vi "Get_Set_Timer_Parameters.vi"(6 "Get/Set":T2, 7 "Element":T3=enum."Current time", 8 "Status/Errors in":refnum<vi>, 9 "Timer parameters in":refnum<vi>, 10 "Value in":u32) -> (0 "Status/Errors out":refnum<vi>, 1 "Timer parameters out":refnum<vi>, 2 "Value out":u32, 3 "Timer cluster":T1={"current time (ms)"=0, "time (ms) screen updated"=0, "time (ms) controls locked"=0, "time (ms) last device check"=0, "time (ms) last data MAS"=0, "time (ms) last data SLV"=0, "time (ms) bad status MAS"=0, "time (ms) bad status SLV"=0, "time (ms) clock error updated"=0, "time delay screen update (ms)"=700, "time delay controls (ms)"=10000, "time delay device check (ms)"=60000, "time until MAS status bad (ms)"=2000, "time until SLV status bad (ms)"=2000, "time until MAS connection bad (ms)"=10000, "time until SLV connection bad (ms)"=10000, "time delay clock error update (ms)"=600000}, 5 "Current time":u32)   [LabVIEW 2013]
uses:
  Controls/Timer_Elements.ctl
  Controls/Get_Set_Timer_Options.ctl
  Controls/Timer_Parameters.ctl
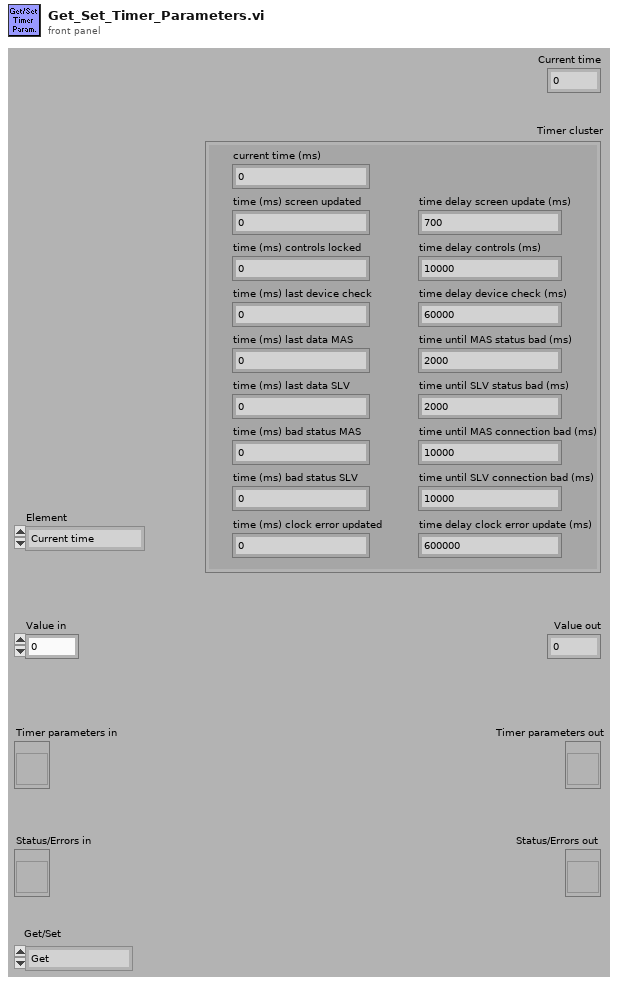
[diagram p1: front panel]
types:
  T1 = typedef "Timer_Parameters.ctl" = cluster{"current time (ms)":u32, "time (ms) screen updated":u32, "time (ms) controls locked":u32, "time (ms) last device check":u32, "time (ms) last data MAS":u32, "time (ms) last data SLV":u32, "time (ms) bad status MAS":u32, "time (ms) bad status SLV":u32, "time (ms) clock error updated":u32, "time delay screen update (ms)":u32, "time delay controls (ms)":u32, "time delay device check (ms)":u32, "time until MAS status bad (ms)":u32, "time until SLV status bad (ms)":u32, "time until MAS connection bad (ms)":u32, "time until SLV connection bad (ms)":u32, "time delay clock error update (ms)":u32}
  T2 = typedef "Get_Set_Timer_Options.ctl" = enum16{"Get", "Get cluster", "Set", "Set to current time"}
  T3 = typedef "Timer_Elements.ctl" = enum16{"Default", "Current time", "Time screen updated", "Time controls locked", "Time last device check", "Time last data MAS", "Time last data SLV", "Time bad status MAS", "Time bad status SLV", "Time clock error updated", "Time delay screen update", "Time delay controls", "Time delay device check", "Time until MAS status bad", "Time until SLV status bad", "Time until MAS connection bad", "Time until SLV connection bad", "Time delay clock error update"}
  T4 = cluster{"current time (ms)":u32, "time (ms) screen updated":u32, "time (ms) controls locked":u32, "time (ms) last device check":u32, "time (ms) last data MAS":u32, "time (ms) last data SLV":u32, "time (ms) bad status MAS":u32, "time (ms) bad status SLV":u32, "time (ms) clock error updated":u32, "time delay screen update (ms)":u32, "time delay controls (ms)":u32, "time delay device check (ms)":u32, "time until MAS status bad (ms)":u32, "time until SLV status bad (ms)":u32, "time until MAS connection bad (ms)":u32, "time until SLV connection bad (ms)":u32, "time delay clock error update (ms)":u32}
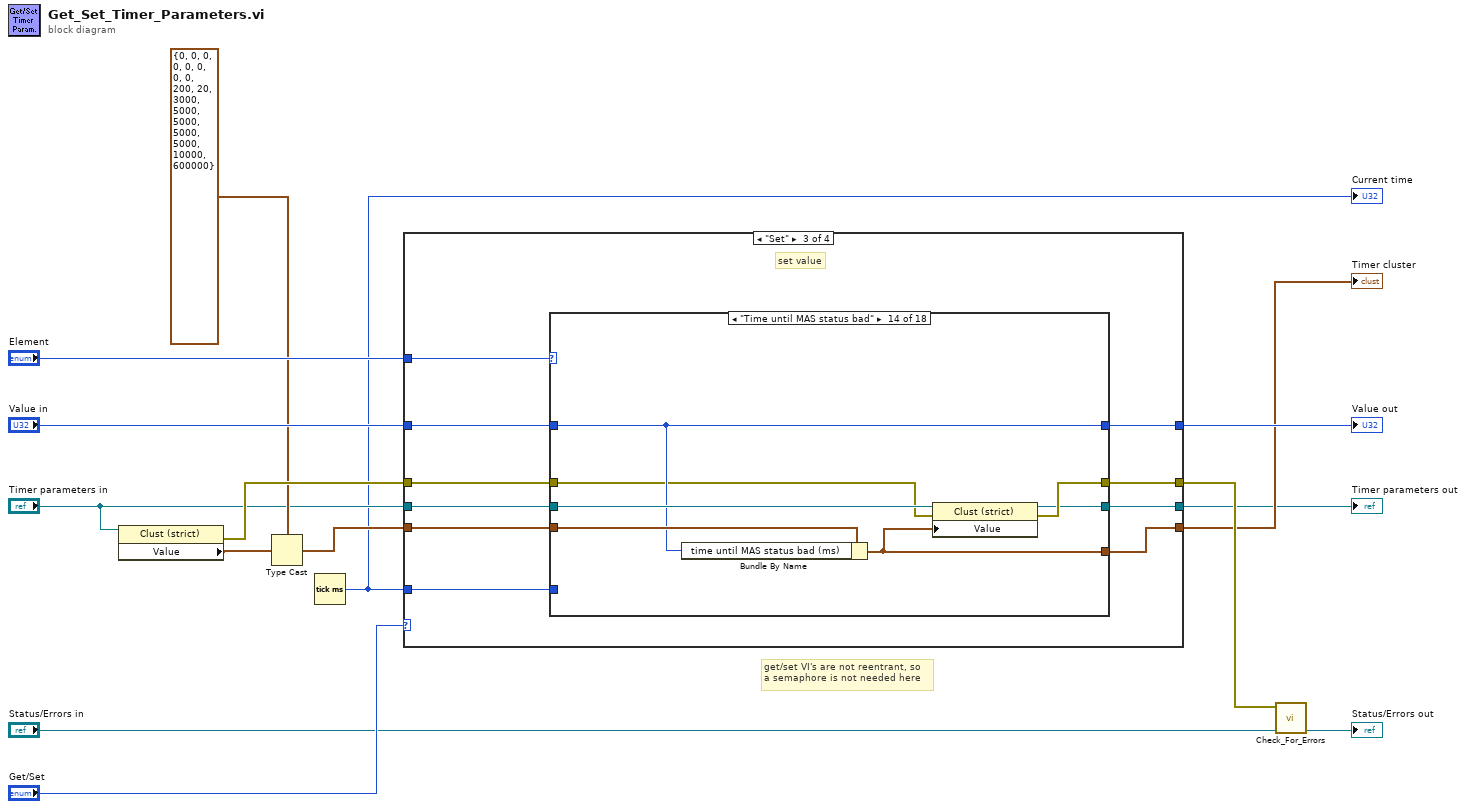
[diagram p0: block diagram]
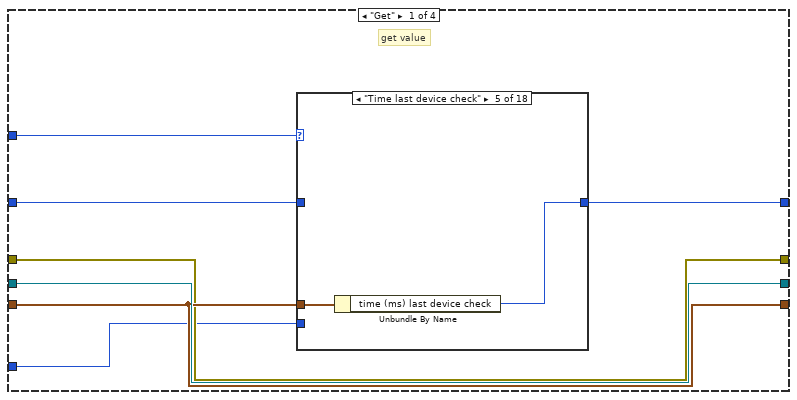
[diagram p2: hidden frame]
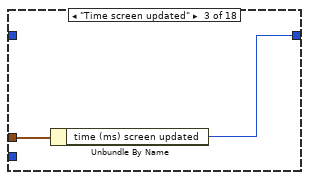
[diagram p5: hidden frame]
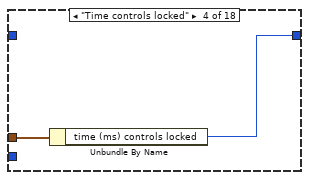
[diagram p6: hidden frame]
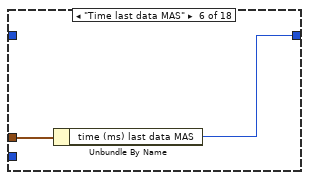
[diagram p7: hidden frame]
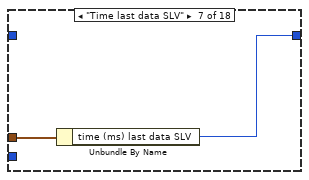
[diagram p8: hidden frame]
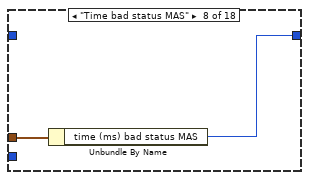
[diagram p9: hidden frame]
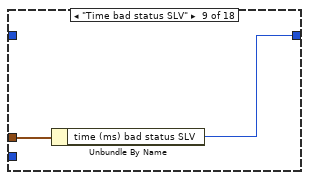
[diagram p10: hidden frame]
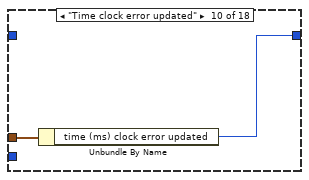
[diagram p11: hidden frame]
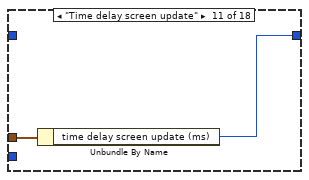
[diagram p12: hidden frame]
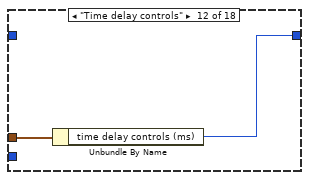
[diagram p13: hidden frame]
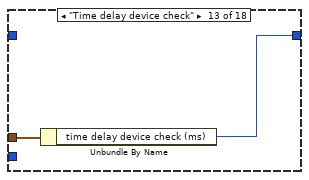
[diagram p14: hidden frame]
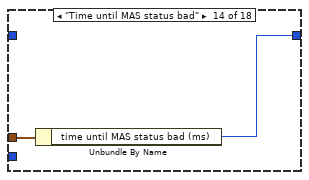
[diagram p15: hidden frame]
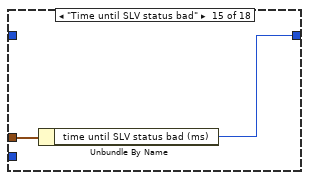
[diagram p16: hidden frame]
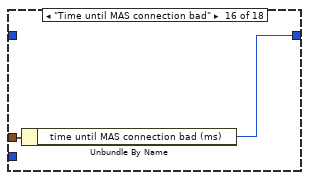
[diagram p17: hidden frame]
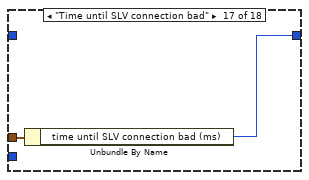
[diagram p18: hidden frame]
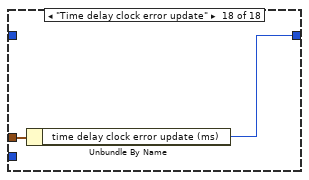
[diagram p19: hidden frame]
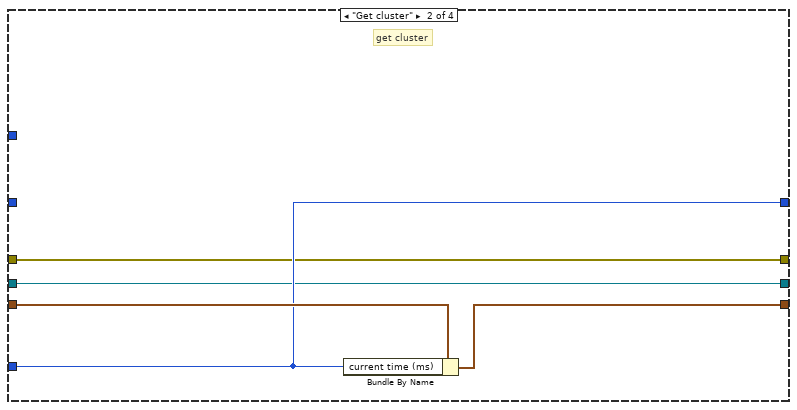
[diagram p20: hidden frame]
diagram:
  # "get/set VI's are not reentrant, so\na semaphore is not needed here"
  n1 = property class="Clust (strict)"(reference="Timer parameters in") -> (error out=w11:errorcluster, "Value"=w6:T4)  [unwired: 1 in, 1 out]
  n2 = Type Cast(type=T1 {"current time (ms)"=0, "time (ms) screen updated"=0, "time (ms) controls locked"=0, "time (ms) last device check"=0, "time (ms) last data MAS"=0, "time (ms) last data SLV"=0, "time (ms) bad status MAS"=0, "time (ms) bad status SLV"=0, "time (ms) clock error updated"=200, "time delay screen update (ms)"=20, "time delay controls (ms)"=3000, "time delay device check (ms)"=5000, "time until MAS status bad (ms)"=5000, "time until SLV status bad (ms)"=5000, "time until MAS connection bad (ms)"=5000, "time until SLV connection bad (ms)"=10000, "time delay clock error update (ms)"=600000} ("Timer parameters"), x=w6) -> (*(type *) &x=w4:T1)
  n3 = Tick Count (ms)() -> (millisecond timer value=w1:u32)
  "Current time" <- w1
  n4 = case shown="\"Set\"" "Get/Set" {
    tunnel: "Element" -> [w22 _ w71 w205]
    tunnel: w4 -> [w18 w61 w65 w204]
    tunnel: "Value in" -> [w19 _ w70 w203]
    tunnel: "Timer parameters in" -> [w20 w58 w69 w202]
    tunnel: [w20 w58 w68 w201] -> w2
    tunnel: [w17 w57 w67 w200] -> w9
    tunnel: [w21 w60 w66 w199] -> w12
    tunnel: [w18 w59 w64 w198] -> w8
    tunnel: w11 -> [w17 w57 w63 w197]
    tunnel: w1 -> [w16 w60 w62 w196]
    frame "Get" {
      # "get value"
      n5 = case shown="\"Time last device check\"" w22 {
        tunnel: w18 -> [_ _ w26 w28 w30 w32 w34 w36 w38 w40 w42 w44 w46 w48 w50 w52 w54 w56]
        tunnel: [w23 w24 w25 w27 w29 w31 w33 w35 w37 w39 w41 w43 w45 w47 w49 w51 w53 w55] -> w21
        tunnel: w19 -> [w23 _ _ _ _ _ _ _ _ _ _ _ _ _ _ _ _ _]
        tunnel: w16 -> [_ w24 _ _ _ _ _ _ _ _ _ _ _ _ _ _ _ _]
        frame Default {
        }
        frame "Current time" {
        }
        frame "Time screen updated" {
          n6 = Unbundle By Name(w26) -> ("time (ms) screen updated"=w25:u32)
        }
        frame "Time controls locked" {
          n7 = Unbundle By Name(w28) -> ("time (ms) controls locked"=w27:u32)
        }
        frame "Time last device check" {
          n8 = Unbundle By Name(w30) -> ("time (ms) last device check"=w29:u32)
        }
        frame "Time last data MAS" {
          n9 = Unbundle By Name(w32) -> ("time (ms) last data MAS"=w31:u32)
        }
        frame "Time last data SLV" {
          n10 = Unbundle By Name(w34) -> ("time (ms) last data SLV"=w33:u32)
        }
        frame "Time bad status MAS" {
          n11 = Unbundle By Name(w36) -> ("time (ms) bad status MAS"=w35:u32)
        }
        frame "Time bad status SLV" {
          n12 = Unbundle By Name(w38) -> ("time (ms) bad status SLV"=w37:u32)
        }
        frame "Time clock error updated" {
          n13 = Unbundle By Name(w40) -> ("time (ms) clock error updated"=w39:u32)
        }
        frame "Time delay screen update" {
          n14 = Unbundle By Name(w42) -> ("time delay screen update (ms)"=w41:u32)
        }
        frame "Time delay controls" {
          n15 = Unbundle By Name(w44) -> ("time delay controls (ms)"=w43:u32)
        }
        frame "Time delay device check" {
          n16 = Unbundle By Name(w46) -> ("time delay device check (ms)"=w45:u32)
        }
        frame "Time until MAS status bad" {
          n17 = Unbundle By Name(w48) -> ("time until MAS status bad (ms)"=w47:u32)
        }
        frame "Time until SLV status bad" {
          n18 = Unbundle By Name(w50) -> ("time until SLV status bad (ms)"=w49:u32)
        }
        frame "Time until MAS connection bad" {
          n19 = Unbundle By Name(w52) -> ("time until MAS connection bad (ms)"=w51:u32)
        }
        frame "Time until SLV connection bad" {
          n20 = Unbundle By Name(w54) -> ("time until SLV connection bad (ms)"=w53:u32)
        }
        frame "Time delay clock error update" {
          n21 = Unbundle By Name(w56) -> ("time delay clock error update (ms)"=w55:u32)
        }
      }
    }
    frame "Get cluster" {
      # "get cluster"
      n22 = Bundle By Name(cluster=w61, "current time (ms)"=w60) -> (w59:T1)
    }
    frame "Set" {
      # "set value"
      n23 = case shown="\"Time until MAS status bad\"" w71 {
        tunnel: w65 -> [w72 w80 w90 w97 w104 w111 w118 w125 w132 w139 w146 w153 w160 w167 w174 w181 w188 w195]
        tunnel: w70 -> [w73 w78 w86 w93 w100 w107 w114 w121 w128 w135 w142 w149 w156 w163 w170 w177 w184 w191]
        tunnel: w63 -> [w74 w79 w85 w92 w99 w106 w113 w120 w127 w134 w141 w148 w155 w162 w169 w176 w183 w190]
        tunnel: w69 -> [w75 w83 w89 w96 w103 w110 w117 w124 w131 w138 w145 w152 w159 w166 w173 w180 w187 w194]
        tunnel: [w75 w81 w88 w94 w101 w108 w115 w122 w129 w136 w143 w150 w157 w164 w171 w178 w185 w192] -> w68
        tunnel: [w74 w82 w87 w95 w102 w109 w116 w123 w130 w137 w144 w151 w158 w165 w172 w179 w186 w193] -> w67
        tunnel: [w73 w78 w86 w93 w100 w107 w114 w121 w128 w135 w142 w149 w156 w163 w170 w177 w184 w191] -> w66
        tunnel: [w72 w77 w84 w91 w98 w105 w112 w119 w126 w133 w140 w147 w154 w161 w168 w175 w182 w189] -> w64
        tunnel: w62 -> [_ w76 _ _ _ _ _ _ _ _ _ _ _ _ _ _ _ _]
        frame Default {
        }
        frame "Current time" {
          n24 = Bundle By Name(cluster=w80, "current time (ms)"=w76) -> (w77:T1)
          n25 = property class="Clust (strict)"(reference=w83, error in=w79, "Value"=w77) -> (reference out=w81:refnum<vi>, error out=w82:errorcluster)
        }
        frame "Time screen updated" {
          n26 = Bundle By Name(cluster=w90, "time (ms) screen updated"=w86) -> (w84:T1)
          n27 = property class="Clust (strict)"(reference=w89, error in=w85, "Value"=w84) -> (reference out=w88:refnum<vi>, error out=w87:errorcluster)
        }
        frame "Time controls locked" {
          n28 = Bundle By Name(cluster=w97, "time (ms) controls locked"=w93) -> (w91:T1)
          n29 = property class="Clust (strict)"(reference=w96, error in=w92, "Value"=w91) -> (reference out=w94:refnum<vi>, error out=w95:errorcluster)
        }
        frame "Time last device check" {
          n30 = Bundle By Name(cluster=w104, "time (ms) last device check"=w100) -> (w98:T1)
          n31 = property class="Clust (strict)"(reference=w103, error in=w99, "Value"=w98) -> (reference out=w101:refnum<vi>, error out=w102:errorcluster)
        }
        frame "Time last data MAS" {
          n32 = Bundle By Name(cluster=w111, "time (ms) last data MAS"=w107) -> (w105:T1)
          n33 = property class="Clust (strict)"(reference=w110, error in=w106, "Value"=w105) -> (reference out=w108:refnum<vi>, error out=w109:errorcluster)
        }
        frame "Time last data SLV" {
          n34 = Bundle By Name(cluster=w118, "time (ms) last data SLV"=w114) -> (w112:T1)
          n35 = property class="Clust (strict)"(reference=w117, error in=w113, "Value"=w112) -> (reference out=w115:refnum<vi>, error out=w116:errorcluster)
        }
        frame "Time bad status MAS" {
          n36 = Bundle By Name(cluster=w125, "time (ms) bad status MAS"=w121) -> (w119:T1)
          n37 = property class="Clust (strict)"(reference=w124, error in=w120, "Value"=w119) -> (reference out=w122:refnum<vi>, error out=w123:errorcluster)
        }
        frame "Time bad status SLV" {
          n38 = Bundle By Name(cluster=w132, "time (ms) bad status SLV"=w128) -> (w126:T1)
          n39 = property class="Clust (strict)"(reference=w131, error in=w127, "Value"=w126) -> (reference out=w129:refnum<vi>, error out=w130:errorcluster)
        }
        frame "Time clock error updated" {
          n40 = Bundle By Name(cluster=w139, "time (ms) clock error updated"=w135) -> (w133:T1)
          n41 = property class="Clust (strict)"(reference=w138, error in=w134, "Value"=w133) -> (reference out=w136:refnum<vi>, error out=w137:errorcluster)
        }
        frame "Time delay screen update" {
          n42 = Bundle By Name(cluster=w146, "time delay screen update (ms)"=w142) -> (w140:T1)
          n43 = property class="Clust (strict)"(reference=w145, error in=w141, "Value"=w140) -> (reference out=w143:refnum<vi>, error out=w144:errorcluster)
        }
        frame "Time delay controls" {
          n44 = Bundle By Name(cluster=w153, "time delay controls (ms)"=w149) -> (w147:T1)
          n45 = property class="Clust (strict)"(reference=w152, error in=w148, "Value"=w147) -> (reference out=w150:refnum<vi>, error out=w151:errorcluster)
        }
        frame "Time delay device check" {
          n46 = Bundle By Name(cluster=w160, "time delay device check (ms)"=w156) -> (w154:T1)
          n47 = property class="Clust (strict)"(reference=w159, error in=w155, "Value"=w154) -> (reference out=w157:refnum<vi>, error out=w158:errorcluster)
        }
        frame "Time until MAS status bad" {
          n48 = Bundle By Name(cluster=w167, "time until MAS status bad (ms)"=w163) -> (w161:T1)
          n49 = property class="Clust (strict)"(reference=w166, error in=w162, "Value"=w161) -> (reference out=w164:refnum<vi>, error out=w165:errorcluster)
        }
        frame "Time until SLV status bad" {
          n50 = Bundle By Name(cluster=w174, "time until SLV status bad (ms)"=w170) -> (w168:T1)
          n51 = property class="Clust (strict)"(reference=w173, error in=w169, "Value"=w168) -> (reference out=w171:refnum<vi>, error out=w172:errorcluster)
        }
        frame "Time until MAS connection bad" {
          n52 = Bundle By Name(cluster=w181, "time until MAS connection bad (ms)"=w177) -> (w175:T1)
          n53 = property class="Clust (strict)"(reference=w180, error in=w176, "Value"=w175) -> (reference out=w178:refnum<vi>, error out=w179:errorcluster)
        }
        frame "Time until SLV connection bad" {
          n54 = Bundle By Name(cluster=w188, "time until SLV connection bad (ms)"=w184) -> (w182:T1)
          n55 = property class="Clust (strict)"(reference=w187, error in=w183, "Value"=w182) -> (reference out=w185:refnum<vi>, error out=w186:errorcluster)
        }
        frame "Time delay clock error update" {
          n56 = Bundle By Name(cluster=w195, "time delay clock error update (ms)"=w191) -> (w189:T1)
          n57 = property class="Clust (strict)"(reference=w194, error in=w190, "Value"=w189) -> (reference out=w192:refnum<vi>, error out=w193:errorcluster)
        }
      }
    }
    frame "Set to current time" {
      # "set value to \"current time\""
      n58 = case shown="Default" w205 {
        tunnel: w204 -> [w207 w211 w216 w223 w230 w237 w244 w251 w258 w265]
        tunnel: w203 -> [_ _ _ _ _ _ _ _ _ _]
        tunnel: w197 -> [w208 w212 w217 w224 w231 w238 w245 w252 w259 w266]
        tunnel: w202 -> [w209 w213 w220 w227 w234 w241 w248 w255 w262 w269]
        tunnel: [w209 w213 w218 w225 w232 w239 w246 w253 w260 w267] -> w201
        tunnel: [w208 w212 w219 w226 w233 w240 w247 w254 w261 w268] -> w200
        tunnel: [w206 w210 w214 w221 w228 w235 w242 w249 w256 w263] -> w199
        tunnel: [w207 w211 w215 w222 w229 w236 w243 w250 w257 w264] -> w198
        tunnel: w196 -> [w206 w210 w214 w221 w228 w235 w242 w249 w256 w263]
        frame Default {
        }
        frame "Current time" {
        }
        frame "Time screen updated" {
          n59 = Bundle By Name(cluster=w216, "time (ms) screen updated"=w214) -> (w215:T1)
          n60 = property class="Clust (strict)"(reference=w220, error in=w217, "Value"=w215) -> (reference out=w218:refnum<vi>, error out=w219:errorcluster)
        }
        frame "Time controls locked" {
          n61 = Bundle By Name(cluster=w223, "time (ms) controls locked"=w221) -> (w222:T1)
          n62 = property class="Clust (strict)"(reference=w227, error in=w224, "Value"=w222) -> (reference out=w225:refnum<vi>, error out=w226:errorcluster)
        }
        frame "Time last device check" {
          n63 = Bundle By Name(cluster=w230, "time (ms) last device check"=w228) -> (w229:T1)
          n64 = property class="Clust (strict)"(reference=w234, error in=w231, "Value"=w229) -> (reference out=w232:refnum<vi>, error out=w233:errorcluster)
        }
        frame "Time last data MAS" {
          n65 = Bundle By Name(cluster=w237, "time (ms) last data MAS"=w235) -> (w236:T1)
          n66 = property class="Clust (strict)"(reference=w241, error in=w238, "Value"=w236) -> (reference out=w239:refnum<vi>, error out=w240:errorcluster)
        }
        frame "Time last data SLV" {
          n67 = Bundle By Name(cluster=w244, "time (ms) last data SLV"=w242) -> (w243:T1)
          n68 = property class="Clust (strict)"(reference=w248, error in=w245, "Value"=w243) -> (reference out=w246:refnum<vi>, error out=w247:errorcluster)
        }
        frame "Time bad status MAS" {
          n69 = Bundle By Name(cluster=w251, "time (ms) bad status MAS"=w249) -> (w250:T1)
          n70 = property class="Clust (strict)"(reference=w255, error in=w252, "Value"=w250) -> (reference out=w253:refnum<vi>, error out=w254:errorcluster)
        }
        frame "Time bad status SLV" {
          n71 = Bundle By Name(cluster=w258, "time (ms) bad status SLV"=w256) -> (w257:T1)
          n72 = property class="Clust (strict)"(reference=w262, error in=w259, "Value"=w257) -> (reference out=w260:refnum<vi>, error out=w261:errorcluster)
        }
        frame "Time clock error updated" {
          n73 = Bundle By Name(cluster=w265, "time (ms) clock error updated"=w263) -> (w264:T1)
          n74 = property class="Clust (strict)"(reference=w269, error in=w266, "Value"=w264) -> (reference out=w267:refnum<vi>, error out=w268:errorcluster)
        }
      }
    }
  }
  "Value out" <- w12
  "Timer cluster" <- w8
  "Timer parameters out" <- w2
  n75 = call "Check_For_Errors.vi"("Status/Errors in"="Status/Errors in", "error in"=w9) -> ("Status/Errors out"=→"Status/Errors out":refnum<vi>)  [unwired: 9 out]
